vi "Find group center (SubVI).vi"(11 "Trap cluster in":T1) -> (2 "Y":sgl, 3 "X":sgl)   [LabVIEW 2012]
uses:
  Trap cluster.ctl
  <vilib>/gmath/NI_Gmath.lvlib
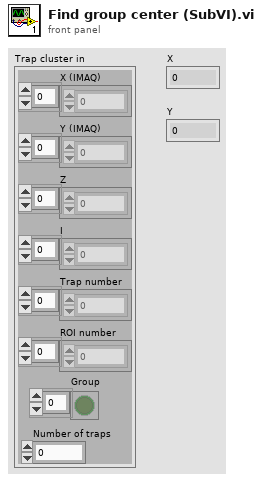
[diagram p1: front panel]
types:
  T1 = typedef "Trap cluster.ctl" = cluster{"X (IMAQ)":sgl[], "Y (IMAQ)":sgl[], "Z":sgl[], "I":sgl[], "Trap number":i32[], "ROI number":i32[], "Number of traps":i32, "Group":bool[]}
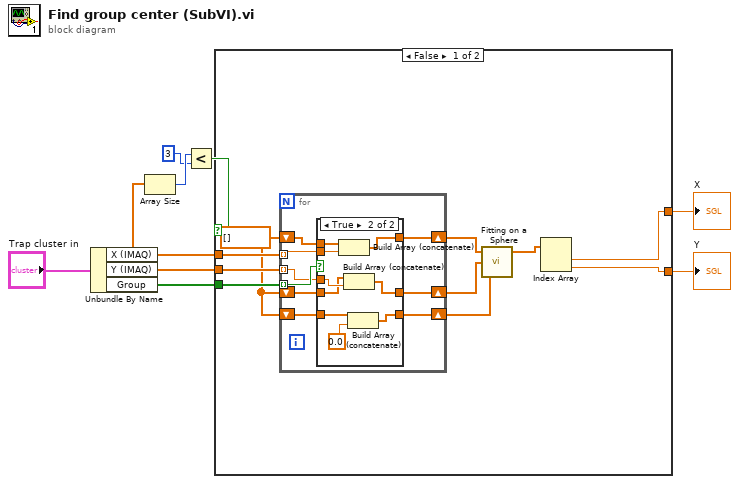
[diagram p0: block diagram]
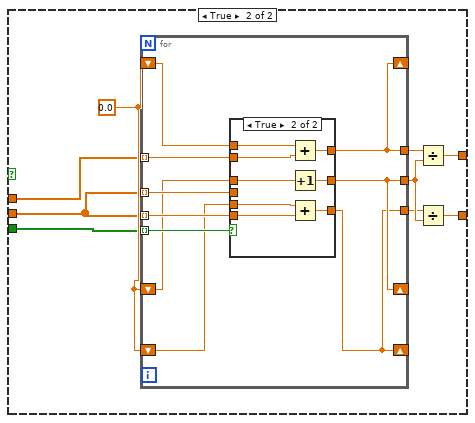
[diagram p3: hidden frame]
diagram:
  n1 = Unbundle By Name("Trap cluster in") -> ("X (IMAQ)"=w4:sgl[], "Y (IMAQ)"=w6:sgl[], "Group"=w5:bool[])
  n2 = Array Size(array=w4) -> (size(s)=w3:i32)
  n3 = Less?(x=w3, y=3 ("x")) -> (x < y?=w1:bool)
  n4 = case shown="False" w1 {
    tunnel: [w10 w48] -> w8
    tunnel: [w11 w47] -> w7
    tunnel: w6 -> [w18 w43]
    tunnel: w5 -> [w17 w42]
    tunnel: w4 -> [w19 w41]
    frame False {
      w16 = sgl[] []
      n5 = for {
        tunnel: w19 -> [w28] mode=indexing
        tunnel: w18 -> [w24] mode=indexing
        tunnel: w17 -> [w25] mode=indexing
        shift-right: [w27] -> w15
        shift-left: w16 -> [w26]
        shift-right: [w23] -> w14
        shift-left: w16 -> [w22]
        shift-right: [w20] -> w13
        shift-left: w16 -> [w21]
        n6 = case shown="True" w25 {
          tunnel: w28 -> [_ w40]
          tunnel: [w31 w39] -> w27
          tunnel: w26 -> [w31 w38]
          tunnel: w24 -> [_ w37]
          tunnel: [w30 w36] -> w23
          tunnel: w22 -> [w30 w35]
          tunnel: w21 -> [w29 w34]
          tunnel: [w29 w33] -> w20
          frame False {
          }
          frame True {
            n7 = Build Array (concatenate)(w38, w40) -> (w39:sgl[])
            n8 = Build Array (concatenate)(w35, w37) -> (w36:sgl[])
            n9 = Build Array (concatenate)(w34, sgl 0.0) -> (w33:sgl[])
          }
        }
      }
      n10 = call <vilib>:"Fitting on a Sphere.vi"("Z"=w13, "Y"=w14, "X"=w15) -> ("x0, y0, z0"=w12:dbl[])  [unwired: 2 out]
      n11 = Index Array(array=w12) -> (element #1=w11:dbl, element #2=w10:dbl)  [unwired: 2 in]
    }
    frame True {
      w49 = sgl 0.0
      n12 = for {
        tunnel: w41 -> [w59] mode=indexing
        tunnel: w43 -> [w58] mode=indexing
        tunnel: w42 -> [w57] mode=indexing
        tunnel: w43 -> [w56] mode=indexing
        tunnel: [w52] -> w46
        tunnel: [w54] -> w44
        tunnel: [w50] -> w45
        shift-right: [w54] -> _
        shift-left: w49 -> [w55]
        shift-right: [w52] -> _
        shift-left: w49 -> [w53]
        shift-right: [w50] -> _
        shift-left: w49 -> [w51]
        n13 = case shown="True" w57 {
          tunnel: w59 -> [_ w70]
          tunnel: w58 -> [_ _]
          tunnel: [w62 w69] -> w54
          tunnel: w55 -> [w62 w68]
          tunnel: [w61 w66] -> w52
          tunnel: w53 -> [w61 w67]
          tunnel: w56 -> [_ w65]
          tunnel: [w60 w64] -> w50
          tunnel: w51 -> [w60 w63]
          frame False {
          }
          frame True {
            n14 = Add(x=w68, y=w70) -> (x+y=w69:sgl)
            n15 = Increment(x=w67) -> (x+1=w66:sgl)
            n16 = Add(x=w63, y=w65) -> (x+y=w64:sgl)
          }
        }
      }
      n17 = Divide(x=w44, y=w46) -> (x/y=w47:sgl)
      n18 = Divide(x=w45, y=w46) -> (x/y=w48:sgl)
    }
  }
  "Y" <- w8
  "X" <- w7
